vi "Magnitude3Dvec.vi"(9 "x 3":dbl, 10 "x in":dbl, 11 "x 1":dbl) -> (3 "sqrt(x)":dbl)   [LabVIEW 2016]
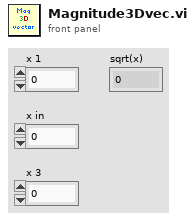
[diagram p1: front panel]
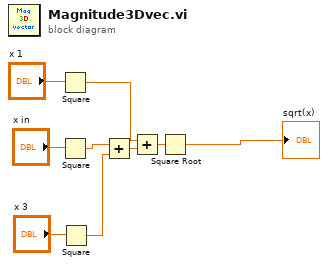
[diagram p0: block diagram]
diagram:
  n1 = Square(x="x 1") -> (x^2=w8:dbl)
  n2 = Square(x="x in") -> (x^2=w2:dbl)
  n3 = Square(x="x 3") -> (x^2=w1:dbl)
  n4 = Add(x=w2, y=w1) -> (x+y=w3:dbl)
  n5 = Add(x=w8, y=w3) -> (x+y=w4:dbl)
  n6 = Square Root(x=w4) -> (sqrt(x)=→"sqrt(x)":dbl)
